vi "generate 96 well rois for cam2.vi"() -> ()   [LabVIEW 2012]
uses:
  <vilib>/vision/NI_Vision_Development_Module.lvlib
panel:
  in  "Save ROI data":path=path "C:/Users/Sleep Box/Desktop/ROI2"
  out "roi data cluster":T1
  in  "Options":T2={"Interpolation Type"=enum."Bilinear Fixed", "Destination Width"=0, "Destination Height"=0, "Fill Value"=0.0}
  in  "Define Corner":bool
  in  "num Y cells":dbl=8.0
  in  "num X cells":dbl=12.0
  in  "three points":dbl[][](array[numeric])=[[86.0, 147.0], [2469.0, 46.0], [2531.0, 1640.0]]
  out "Image":T3(plugin-control)
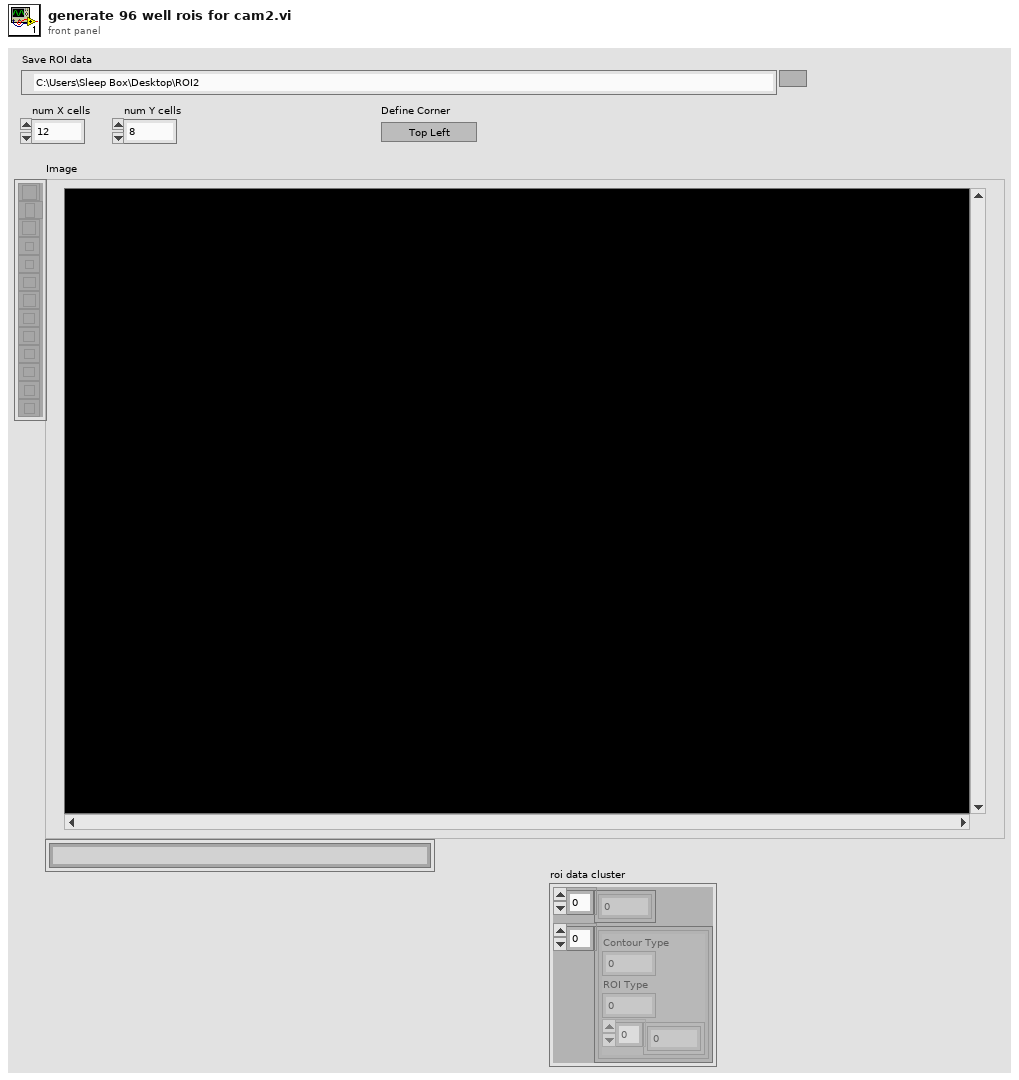
[diagram p1: front panel]
types:
  T1 = cluster{i32[], cluster{"Contour Type":u32, "ROI Type":u32, i32[]}[]}
  T2 = cluster{"Interpolation Type":enum32{"Zero Order", "Bilinear", "Quadratic", "Cubic", "Bilinear Fixed"}, "Destination Width":u32, "Destination Height":u32, "Fill Value":sgl}
  T3 = typedef "IMAQ Image.ctl" = refnum<image>
  T4 = enum16{"open", "replace", "create", "open or create", "replace or create", "replace or create with confirmation"}
  T5 = cluster{"Global Rectangle":i32[], "Contours":cluster{"Contour Type":u32, "ROI Type":u32, "Points":i32[]}[]}
  T6 = cluster{"Contour Type":u32, "ROI Type":u32, "Points":i32[]}[]
  T7 = cluster{"Contour Type":u32, "ROI Type":u32, "Points":i32[]}
  T8 = cluster{"Contour Type":u32, "ROI Type":u32, i32[]}
  T9 = cluster{"Contour Type":u32, "ROI Type":u32, i32[]}[]
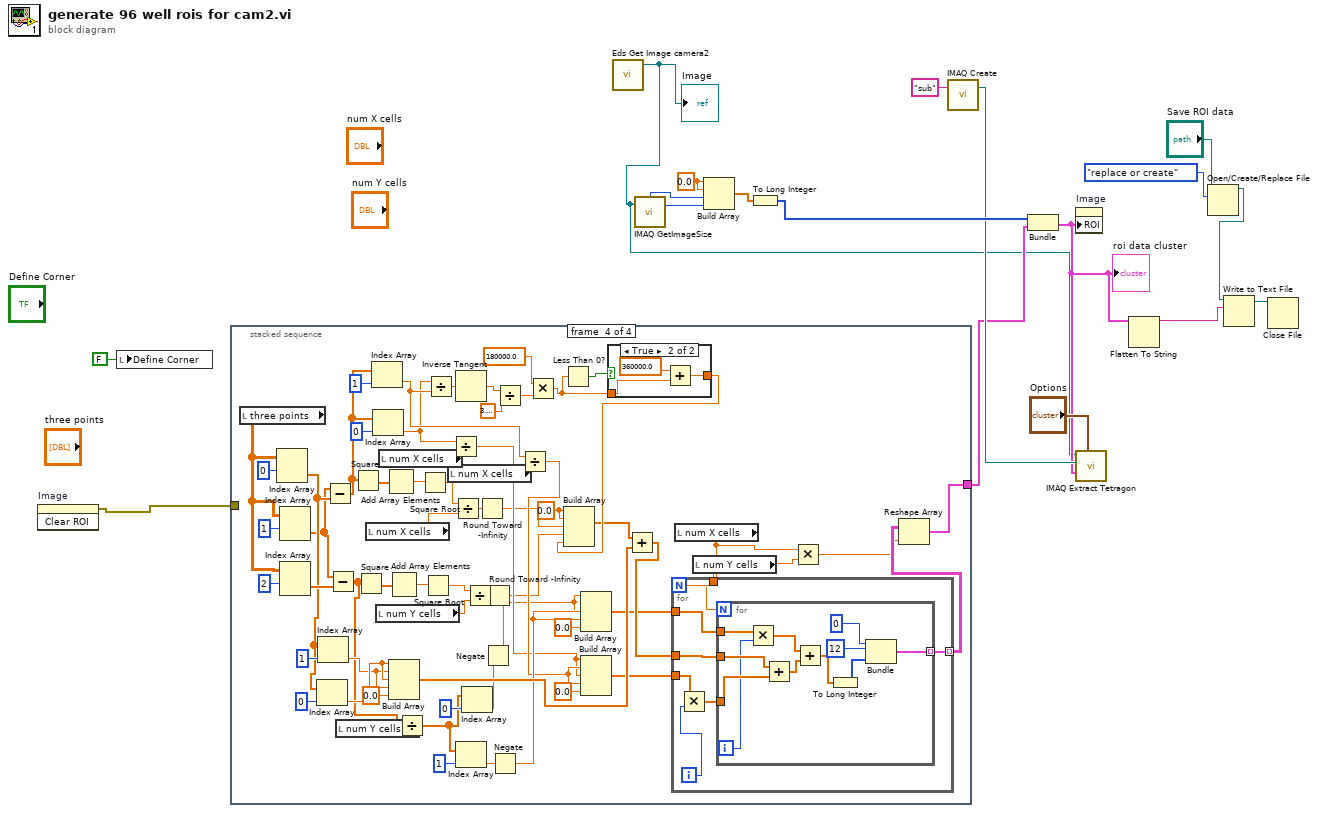
[diagram p0: block diagram]
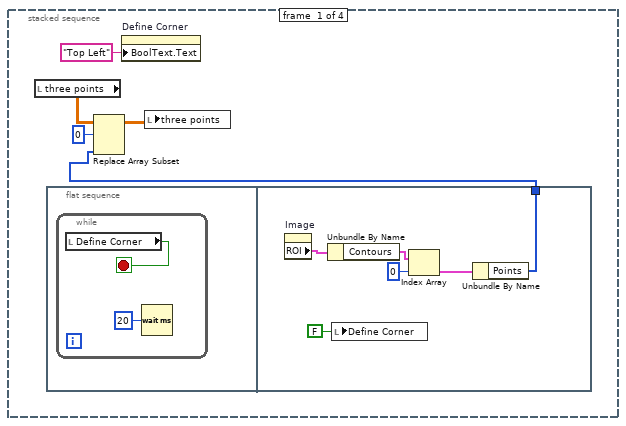
[diagram p2: hidden frame]
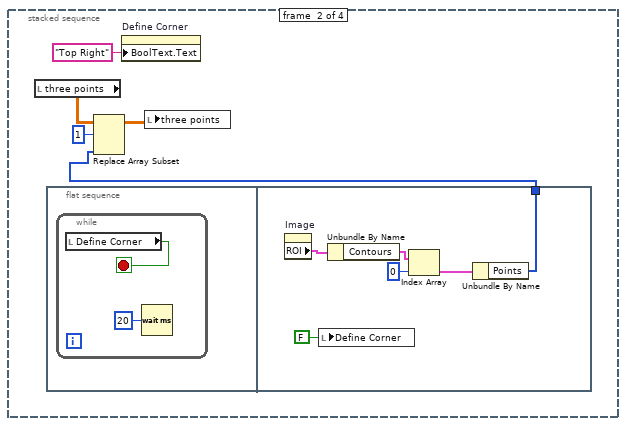
[diagram p3: hidden frame]
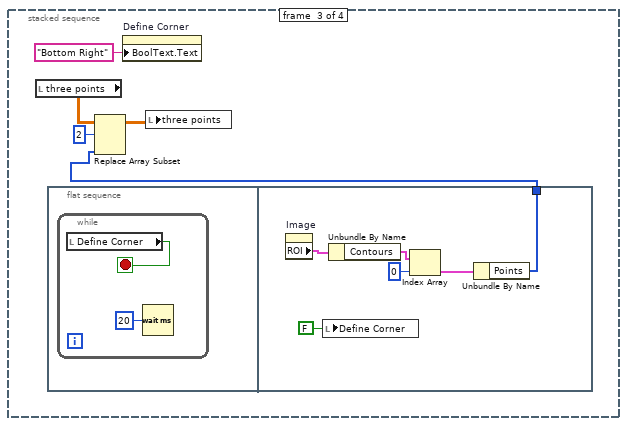
[diagram p4: hidden frame]
diagram:
  w17 = 0.0 ("element")
  n1 = invoke on="Image" class="ImageControl" method="Clear ROI"() -> (error out=w18:errorcluster)  [unwired: 3 in, 2 out]
  n2 = local write "Define Corner"(FALSE ("Define Corner")) -> ()
  n3 = stacked-sequence {
    tunnel: [_ _ _ w84] -> w8
    tunnel: w18 -> [_ _ _ _]
    frame #0 {
      n4 = local read "three points"() -> (w21:dbl[][])
      n5 = flat-sequence {
        tunnel: [w27] -> w22
        frame #0 {
          n6 = while {
            stop <- w25 stop-if-true
            n7 = local read "Define Corner"() -> (w25:bool)
            n8 = Wait (ms)(milliseconds to wait=u32 20) -> ()  [unwired: 1 out]
          }
        }
        frame #1 {
          n9 = property on="Image" class="ImageControl"() -> ("ROI"=w31:T5)  [unwired: 2 in, 2 out]
          n10 = Unbundle By Name(w31) -> ("Contours"=w30:T6)
          n11 = local write "Define Corner"(FALSE ("Define Corner")) -> ()
          n12 = Index Array(array=w30, index=0) -> (element=w28:T7)
          n13 = Unbundle By Name(w28) -> ("Points"=w27:i32[])
        }
      }
      n14 = Replace Array Subset(array=w21, new element=w22, index (row)=0) -> (w20:dbl[][])  [unwired: 1 in]
      n15 = property on="Define Corner" class="Bool (strict)"("BoolText.Text"="Top Left" ("Boolean Text.Text")) -> ()  [unwired: 2 in, 2 out]
      n16 = local write "three points"(w20) -> ()
    }
    frame #1 {
      n17 = local read "three points"() -> (w34:dbl[][])
      n18 = flat-sequence {
        tunnel: [w40] -> w35
        frame #0 {
          n19 = while {
            stop <- w38 stop-if-true
            n20 = local read "Define Corner"() -> (w38:bool)
            n21 = Wait (ms)(milliseconds to wait=u32 20) -> ()  [unwired: 1 out]
          }
        }
        frame #1 {
          n22 = property on="Image" class="ImageControl"() -> ("ROI"=w44:T5)  [unwired: 2 in, 2 out]
          n23 = local write "Define Corner"(FALSE ("Define Corner")) -> ()
          n24 = Unbundle By Name(w44) -> ("Contours"=w43:T6)
          n25 = Index Array(array=w43, index=0) -> (element=w41:T7)
          n26 = Unbundle By Name(w41) -> ("Points"=w40:i32[])
        }
      }
      n27 = Replace Array Subset(array=w34, new element=w35, index (row)=1) -> (w33:dbl[][])  [unwired: 1 in]
      n28 = property on="Define Corner" class="Bool (strict)"("BoolText.Text"="Top Right" ("Boolean Text.Text")) -> ()  [unwired: 2 in, 2 out]
      n29 = local write "three points"(w33) -> ()
    }
    frame #2 {
      n30 = local read "three points"() -> (w47:dbl[][])
      n31 = flat-sequence {
        tunnel: [w53] -> w48
        frame #0 {
          n32 = while {
            stop <- w51 stop-if-true
            n33 = local read "Define Corner"() -> (w51:bool)
            n34 = Wait (ms)(milliseconds to wait=u32 20) -> ()  [unwired: 1 out]
          }
        }
        frame #1 {
          n35 = property on="Image" class="ImageControl"() -> ("ROI"=w57:T5)  [unwired: 2 in, 2 out]
          n36 = local write "Define Corner"(FALSE ("Define Corner")) -> ()
          n37 = Unbundle By Name(w57) -> ("Contours"=w56:T6)
          n38 = Index Array(array=w56, index=0) -> (element=w54:T7)
          n39 = Unbundle By Name(w54) -> ("Points"=w53:i32[])
        }
      }
      n40 = Replace Array Subset(array=w47, new element=w48, index (row)=2) -> (w46:dbl[][])  [unwired: 1 in]
      n41 = property on="Define Corner" class="Bool (strict)"("BoolText.Text"="Bottom Right" ("Boolean Text.Text")) -> ()  [unwired: 2 in, 2 out]
      n42 = local write "three points"(w46) -> ()
    }
    frame #3 {
      w94 = 0.0 ("element")
      n43 = local read "three points"() -> (w65:dbl[][])
      n44 = Index Array(array=w65, index (row)=0) -> (element=w83:dbl[])  [unwired: 1 in]
      n45 = Index Array(array=w65, index (row)=1) -> (element=w82:dbl[])  [unwired: 1 in]
      n46 = Index Array(array=w65, index (row)=2) -> (element=w113:dbl[])  [unwired: 1 in]
      n47 = Index Array(array=w83, index=0) -> (element=w93:dbl)
      n48 = Index Array(array=w83, index=1) -> (element=w92:dbl)
      n49 = Subtract(x=w82, y=w83) -> (x-y=w106:dbl[])
      n50 = Subtract(x=w82, y=w113) -> (x-y=w79:dbl[])
      n51 = local read "num Y cells"() -> (w97:dbl)
      n52 = Square(x=w106) -> (x^2=w118:dbl[])
      n53 = Square(x=w79) -> (x^2=w114:dbl[])
      n54 = local read "num X cells"() -> (w112:dbl)
      n55 = Index Array(array=w106, index=1) -> (element=w63:dbl)
      n56 = Index Array(array=w106, index=0) -> (element=w62:dbl)
      n57 = local read "num Y cells"() -> (w110:dbl)
      n58 = local read "num X cells"() -> (w98:dbl)
      n59 = Add Array Elements(numeric array=w118) -> (sum=w117:dbl)
      n60 = Add Array Elements(numeric array=w114) -> (sum=w115:dbl)
      n61 = Build Array(w93, w92, w93, w92, 0.0 ("element")) -> (w90:dbl[])
      n62 = Divide(x=w79, y=w97) -> (x/y=w76:dbl[])
      n63 = Square Root(x=w117) -> (sqrt(x)=w99:dbl)
      n64 = Square Root(x=w115) -> (sqrt(x)=w111:dbl)
      n65 = Divide(x=w62, y=w63) -> (x/y=w66:dbl)
      n66 = local read "num X cells"() -> (w74:dbl)
      n67 = Divide(x=w62, y=w98) -> (x/y=w72:dbl)
      n68 = Divide(x=w99, y=w112) -> (x/y=w101:dbl)
      n69 = Inverse Tangent(1:w66) -> (0:w67:dbl)
      n70 = Index Array(array=w76, index=1) -> (element=w80:dbl)
      n71 = Index Array(array=w76, index=0) -> (element=w75:dbl)
      n72 = Divide(x=w111, y=w110) -> (x/y=w100:dbl)
      n73 = Round Toward -Infinity(1:w101) -> (0:w59:dbl)
      n74 = Negate(x=w75) -> (-x=w71:dbl)
      n75 = Round Toward -Infinity(1:w100) -> (0:w58:dbl)
      n76 = Negate(x=w80) -> (-x=w78:dbl)
      n77 = Divide(x=w67, y=3.141592653589793) -> (x/y=w64:dbl)
      n78 = Divide(x=w63, y=w74) -> (x/y=w73:dbl)
      n79 = Multiply(x=180000.0, y=w64) -> (x*y=w103:dbl)
      n80 = Less Than 0?(x=w103) -> (x < 0?=w104:bool)
      n81 = Build Array(w71, w78, w71, w78, 0.0 ("element")) -> (w86:dbl[])
      n82 = Build Array(w72, w73, w72, w73, 0.0 ("element")) -> (w87:dbl[])
      n83 = case shown="True" w104 {
        tunnel: w103 -> [w139 w141]
        tunnel: [w139 w140] -> w102
        frame False {
        }
        frame True {
          n84 = Add(x=360000.0, y=w141) -> (x+y=w140:dbl)
        }
      }
      n85 = Build Array(w94, w94, w59, w58, w102) -> (w89:dbl[])
      n86 = Add(x=w89, y=w90) -> (x+y=w88:dbl[])
      n87 = local read "num X cells"() -> (w70:dbl)
      n88 = local read "num Y cells"() -> (w69:dbl)
      n89 = for {
        N: w70 -> [_]
        tunnel: w69 -> [w127]
        tunnel: w88 -> [w126]
        tunnel: w87 -> [w124]
        tunnel: w86 -> [w125]
        tunnel: [w121] -> w85 mode=indexing
        i -> [w123]
        n90 = Multiply(x=w124, y=w123) -> (x*y=w122:dbl[])
        n91 = for {
          N: w127 -> [_]
          tunnel: w126 -> [w135]
          tunnel: w125 -> [w133]
          tunnel: w122 -> [w134]
          tunnel: [w128] -> w121 mode=indexing
          i -> [w132]
          n92 = Multiply(x=w133, y=w132) -> (x*y=w129:dbl[])
          n93 = Add(x=w135, y=w134) -> (x+y=w130:dbl[])
          n94 = Add(x=w129, y=w130) -> (x+y=w131:dbl[])
          n95 = To Long Integer(number=w131) -> (32bit integer=w136:i32[])
          n96 = Bundle("Contour Type"=u32 0, "ROI Type"=u32 12, w136) -> (w128:T8)  [unwired: 1 in]
        }
      }
      n97 = Multiply(x=w70, y=w69) -> (x*y=w68:dbl)
      n98 = Reshape Array(w85, w68) -> (w84:T9)
    }
  }
  n99 = call "Eds Get Image camera2.vi"() -> ("Image"=w1:T3)  [unwired: 5 in]
  "Image" <- w1
  n100 = call "IMAQ GetImageSize"("Image"=w1) -> ("Y Resolution"=w15:i32, "X Resolution"=w16:i32)  [unwired: 3 in, 1 out]
  n101 = Build Array(w17, w17, w16, w15) -> (w14:dbl[])
  n102 = To Long Integer(number=w14) -> (32bit integer=w13:i32[])
  n103 = call "IMAQ Create"("Image Name"="sub") -> ("New Image"=w10:T3)  [unwired: 4 in, 1 out]
  n104 = Bundle(w13, w8) -> (w7:T1)  [unwired: 1 in]
  "roi data cluster" <- w7
  n105 = property on="Image" class="ImageControl"("ROI"=w7) -> ()  [unwired: 2 in, 2 out]
  n106 = call-poly "IMAQ Extract Tetragon"("Options"="Options", "ROI Descriptor"=w7, "Image Dst"=w10, "Image Src"=w1) -> ()  [unwired: 6 in, 2 out]
  n107 = Flatten To String(anything=w7) -> (data string=w3:string)  [unwired: 3 in, 2 out]
  n108 = Open/Create/Replace File(file path (use dialog)="Save ROI data", operation (0:open)=T4."replace or create") -> (refnum out=w4:refnum<file>)  [unwired: 4 in, 2 out]
  n109 = Write to Text File(file (use dialog)=w4, text=w3) -> (refnum out=w2:refnum<file>)  [unwired: 2 in, 2 out]
  n110 = Close File(refnum=w2) -> ()  [unwired: 1 in, 2 out]
